vi "Scalar and Compound Data with Attributes.vi"() -> ()   [LabVIEW 2011]
panel:
  in  "my_scalar":T1(array[cluster])=[{"#attributes"={"foo"="bar 1"}, "my_scalar"=1.0}, {"#attributes"={"foo"="bar 2"}, "my_scalar"=2.0}]
  out "XML String":string="<my_scalar foo=\"bar 1\">1</my_scalar>\r\n<my_scalar foo=\"bar 2\">2</my_scalar>"
  in  "my_scalar":dbl=2.0
  out "XML String":string="<my_scalar>2</my_scalar>"
  in  "my_scalar":T2={"#attributes"={"foo"="a"}, "my_scalar"=2.0}
  out "XML String":string="<my_scalar foo=\"a\">2</my_scalar>"
  in  "my_compound_data":cluster{"element":string[]}={"element"=["red", "green", "blue"]}
  out "XML String":string="<my_compound_data>\r\n  <element>red</element>\r\n  <element>green</element>\r\n  <element>blue</element>\r\n</my_compound_data>"
  out "XML String":string="<my_compound_data>\r\n  <element_1>hello</element_1>\r\n  <element_2>2</element_2>\r\n</my_compound_data>"
  in  "my_compound_data":cluster{"element_1":string, "element_2":dbl}={"element_1"="hello", "element_2"=2.0}
  in  "my_compound_data":T3={"#attributes"={"attribute_1"="a"}, "element_1"="hello", "element_2"=2.0}
  out "XML String":string="<my_compound_data attribute_1=\"a\">\r\n  <element_1>hello</element_1>\r\n  <element_2>2</element_2>\r\n</my_compound_data>"
  # "Compound Element (dissimilar-named child elements)"
  # "Scalar Element"
  # "Scalar Element with Attributes"
  # "Compound Element (like-named child elements)"
  # "same name"
  # "one child"
  # "List of Scalar Elements with Attributes"
  # "Compound Elements with Attributes"
  # "same name"
  # "one child"
  # "array element names are always ignored"
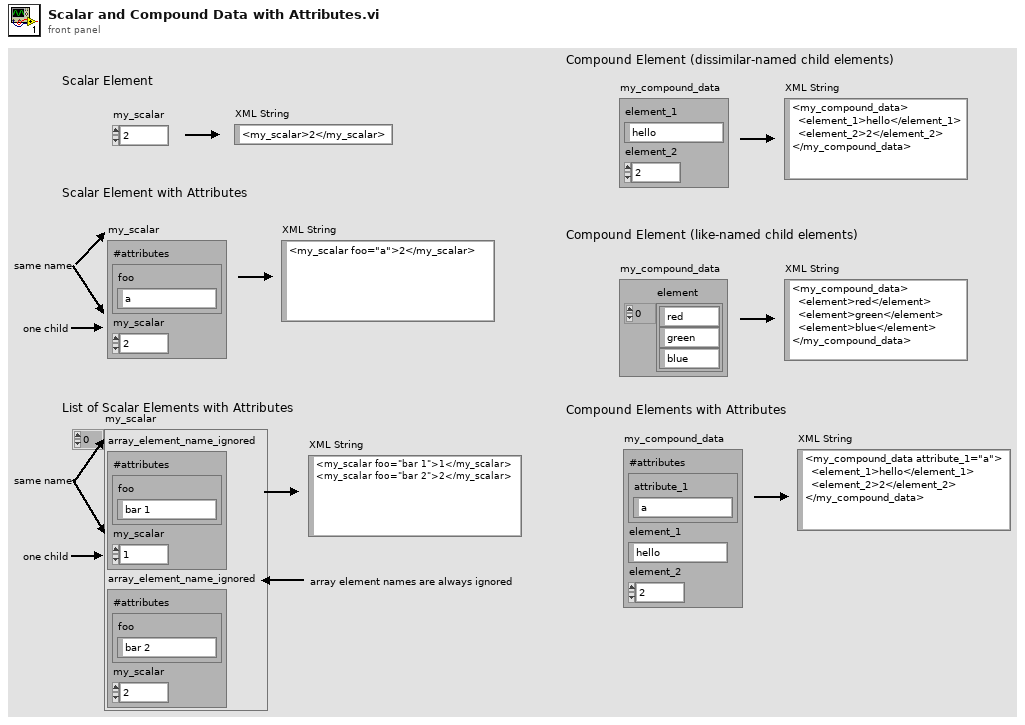
[diagram p1: front panel]
types:
  T1 = cluster{"#attributes":cluster{"foo":string}, "my_scalar":dbl}[]
  T2 = cluster{"#attributes":cluster{"foo":string}, "my_scalar":dbl}
  T3 = cluster{"#attributes":cluster{"attribute_1":string}, "element_1":string, "element_2":dbl}
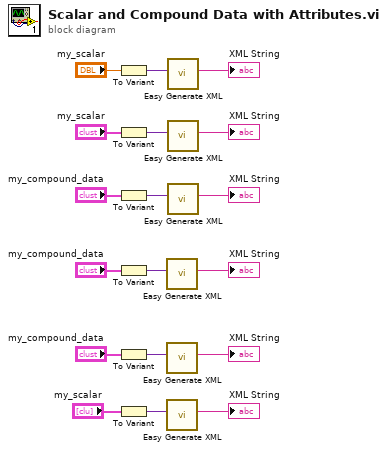
[diagram p0: block diagram]
diagram:
  n1 = To Variant(anything="my_scalar") -> (Variant=w4:variant)
  n2 = To Variant(anything="my_scalar") -> (Variant=w5:variant)
  n3 = To Variant(anything="my_compound_data") -> (Variant=w6:variant)
  n4 = To Variant(anything="my_compound_data") -> (Variant=w14:variant)
  n5 = To Variant(anything="my_compound_data") -> (Variant=w13:variant)
  n6 = To Variant(anything="my_scalar") -> (Variant=w3:variant)
  n7 = call "Easy Generate XML.vi"("LabVIEW Data"=w14) -> ("XML String"=→"XML String":string)  [unwired: 9 in, 1 out]
  n8 = call "Easy Generate XML.vi"("LabVIEW Data"=w13) -> ("XML String"=→"XML String":string)  [unwired: 9 in, 1 out]
  n9 = call "Easy Generate XML.vi"("LabVIEW Data"=w3) -> ("XML String"=→"XML String":string)  [unwired: 9 in, 1 out]
  n10 = call "Easy Generate XML.vi"("LabVIEW Data"=w4) -> ("XML String"=→"XML String":string)  [unwired: 9 in, 1 out]
  n11 = call "Easy Generate XML.vi"("LabVIEW Data"=w5) -> ("XML String"=→"XML String":string)  [unwired: 9 in, 1 out]
  n12 = call "Easy Generate XML.vi"("LabVIEW Data"=w6) -> ("XML String"=→"XML String":string)  [unwired: 9 in, 1 out]
